vi "Data_Packet_to_Processed_Bytes.vi"(0 "Data Packet In":T1, 1 "error in (no error)":errorcluster) -> (2 "Data Packet Out":T1, 3 "Processed Bytes":u8[](array[numeric]), 4 "error out":errorcluster)   [LabVIEW 2017]
uses:
  Packet.ctl
  Packet_Direction.ctl
  Packet_Type.ctl
  Packet_Priority.ctl
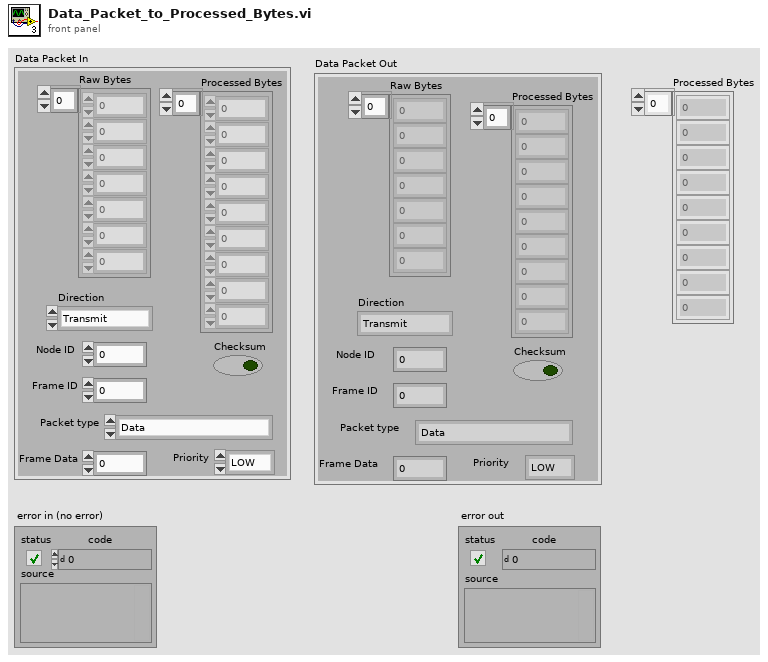
[diagram p1: front panel]
types:
  T1 = typedef "Packet.ctl" = cluster{"Raw Bytes":u8[], "Checksum":bool, "Direction":T2, "Processed Bytes":u8[], "Node ID":u8, "Packet type":T3, "Frame Data":u32, "Priority":T4, "Frame ID":u8}
  T2 = typedef "Packet_Direction.ctl" = enum16{"Transmit", "Receive", "Bidirectional"}
  T3 = typedef "Packet_Type.ctl" = enum16{"Data", "Connection Management", "Remote Request", "Error/Status"}
  T4 = typedef "Packet_Priority.ctl" = enum16{"LOW", "HIGH"}
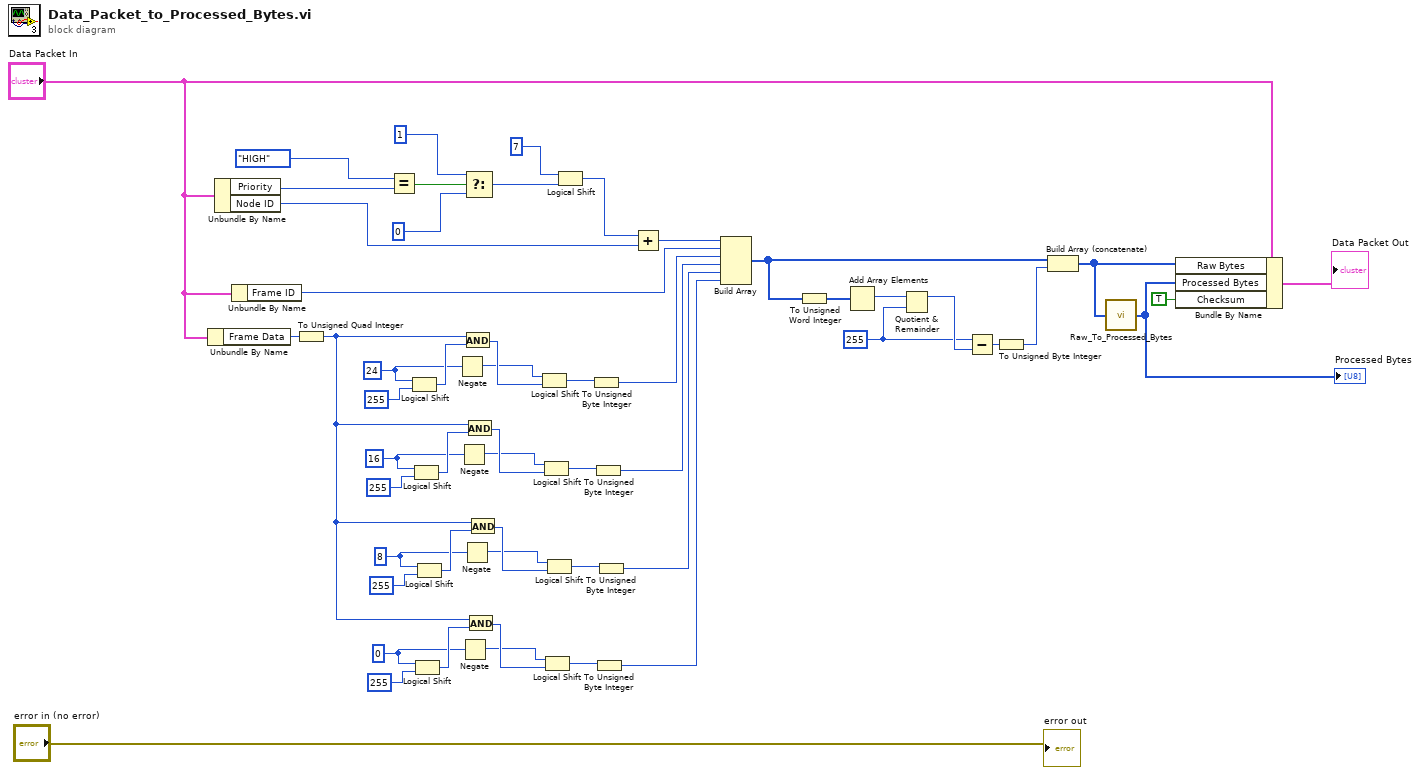
[diagram p0: block diagram]
diagram:
  w10 = u16 255 ("y")
  w21 = i16 0 ("y")
  w27 = i16 8 ("y")
  w33 = i16 16 ("y")
  w39 = i16 24 ("y")
  n1 = Unbundle By Name("Data Packet In") -> ("Frame Data"=w43:u32)
  n2 = Unbundle By Name("Data Packet In") -> ("Priority"=w54:T4, "Node ID"=w46:u8)
  n3 = Unbundle By Name("Data Packet In") -> ("Frame ID"=w44:u8)
  n4 = To Unsigned Quad Integer(1:w43) -> (0:w18:u64)
  n5 = Equal?(x=Packet_Priority."HIGH", y=w54) -> (x = y?=w52:bool)
  n6 = Logical Shift(y=w39, x=u64 255 ("y")) -> (x << y=w41:u64)
  n7 = Logical Shift(y=w33, x=u64 255 ("y")) -> (x << y=w35:u64)
  n8 = Logical Shift(y=w21, x=u64 255 ("y")) -> (x << y=w23:u64)
  n9 = Logical Shift(y=w27, x=u64 255 ("y")) -> (x << y=w29:u64)
  n10 = Negate(x=w39) -> (-x=w38:i16)
  n11 = Negate(x=w33) -> (-x=w32:i16)
  n12 = Negate(x=w21) -> (-x=w20:i16)
  n13 = Negate(x=w27) -> (-x=w26:i16)
  n14 = And(x=w18, y=w41) -> (x .and. y?=w40:u64)
  n15 = Select(t=u8 1, s=w52, f=u8 0) -> (s? t:f=w49:u8)
  n16 = And(x=w18, y=w35) -> (x .and. y?=w34:u64)
  n17 = And(x=w18, y=w23) -> (x .and. y?=w22:u64)
  n18 = And(x=w18, y=w29) -> (x .and. y?=w28:u64)
  n19 = Logical Shift(y=w38, x=w40) -> (x << y=w37:u64)
  n20 = Logical Shift(y=w32, x=w34) -> (x << y=w31:u64)
  n21 = Logical Shift(y=w20, x=w22) -> (x << y=w19:u64)
  n22 = Logical Shift(y=w26, x=w28) -> (x << y=w25:u64)
  n23 = Logical Shift(y=i16 7, x=w49) -> (x << y=w47:u8)
  n24 = To Unsigned Byte Integer(number=w37) -> (unsigned 8bit integer=w17:u8)
  n25 = To Unsigned Byte Integer(number=w31) -> (unsigned 8bit integer=w16:u8)
  n26 = To Unsigned Byte Integer(number=w19) -> (unsigned 8bit integer=w14:u8)
  n27 = To Unsigned Byte Integer(number=w25) -> (unsigned 8bit integer=w15:u8)
  n28 = Add(x=w47, y=w46) -> (x+y=w45:u8)
  n29 = Build Array(w45, w44, w17, w16, w15, w14) -> (w9:u8[])
  n30 = To Unsigned Word Integer(number=w9) -> (unsigned 16bit integer=w13:u16[])
  n31 = Add Array Elements(numeric array=w13) -> (sum=w12:u16)
  n32 = Quotient & Remainder(x=w12, y=w10) -> (x-y*floor(x/y)=w11:u16)  [unwired: 1 out]
  n33 = Subtract(x=w10, y=w11) -> (x-y=w8:u16)
  n34 = To Unsigned Byte Integer(number=w8) -> (unsigned 8bit integer=w6:u8)
  n35 = Build Array (concatenate)(w9, w6) -> (w3:u8[])
  n36 = call "Raw_To_Processed_Bytes.vi"("Raw Bytes"=w3) -> ("Processed Bytes"=w2:u8[])
  "Processed Bytes" <- w2
  n37 = Bundle By Name(cluster="Data Packet In", "Raw Bytes"=w3, "Processed Bytes"=w2, "Checksum"=TRUE) -> (→"Data Packet Out":T1)
  "error out" <- "error in (no error)"
